vi "belt_timing.vi"(4 "time (ms)":i32, 5 "Loop ID":i32) -> (1 "finished?":bool)   [LabVIEW 2011]
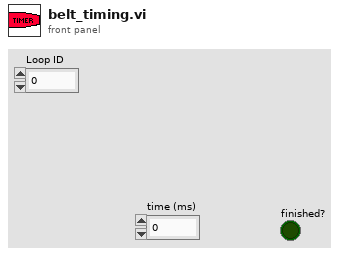
[diagram p1: front panel]
types:
  T1 = typedef "subStates.ctl" = enum16{"null", "wait", "driver control", "auto", "manual override", "autoDrive", "hold position", "rotate", "end"}
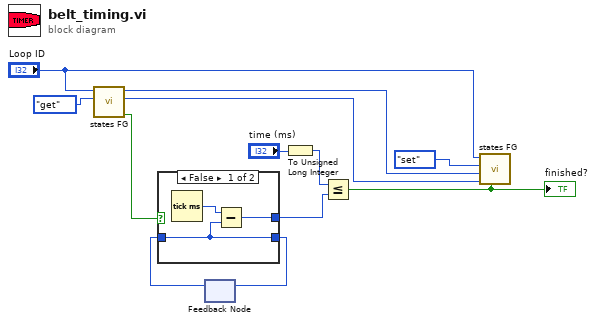
[diagram p0: block diagram]
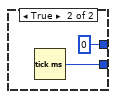
[diagram p2: hidden frame]
diagram:
  n1 = call "states FG.vi"("menu (get)"=enum16{"set", "get"}."get", "Loop ID"="Loop ID") -> ("first call?"=w11:bool, "state # out"=w4:i32, "subState out"=w5:T1)  [unwired: 6 in, 1 out]
  n2 = feedback #1() -> (w9:u32)  [unwired: 1 in]
  n3 = case shown="False" w11 {
    tunnel: [w14 w17] -> w10
    tunnel: w9 -> [w14 _]
    tunnel: [w13 u32 0] -> w8
    frame False {
      n4 = Tick Count (ms)() -> (millisecond timer value=w15:u32)
      n5 = Subtract(x=w15, y=w14) -> (x-y=w13:u32)
    }
    frame True {
      n6 = Tick Count (ms)() -> (millisecond timer value=w17:u32)
    }
  }
  n7 = feedback-in #1(w10) -> ()
  n8 = To Unsigned Long Integer(number="time (ms)") -> (unsigned 32bit integer=w6:u32)
  n9 = Less Or Equal?(x=w6, y=w8) -> (x <= y?=w1:bool)
  "finished?" <- w1
  n10 = call "states FG.vi"("exit in"=w1, "state # in"=w4, "subState in"=w5, "menu (get)"=enum16{"set", "get"}."set", "Loop ID"="Loop ID") -> ()  [unwired: 3 in, 4 out]
